vi "Get SMO HELP.vi"(8 "error in (no error)":errorcluster, 10 "Command":string, 11 "Instrument in":refnum<class "Instrument.lvclass">) -> (0 "error out":errorcluster, 2 "output cluster":T1, 3 "Instrument out":refnum<class "Instrument.lvclass">)   [LabVIEW 2019, in "Instrument.lvclass"]
uses:
  Instrument.lvclass
  Help/typedefs/Help--cluster.ctl
  Typedefs/Instrument.Commands--Enum.ctl
  Typedefs/Instrument.IDN--cluster.ctl
  Help/Help.lvclass
  <vilib>/JKI/JKI SMO/SMO/SMO.lvclass
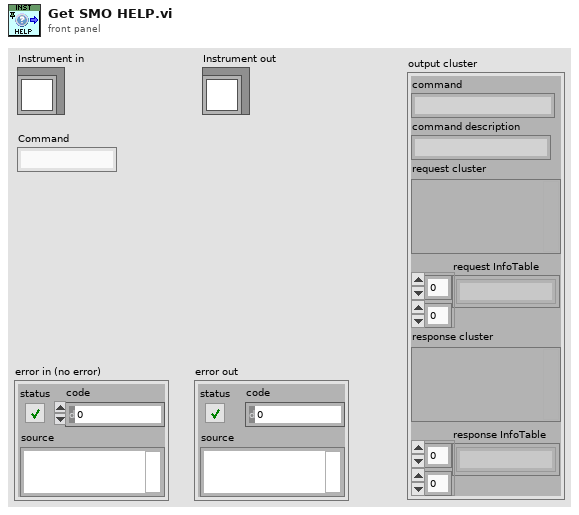
[diagram p1: front panel]
types:
  T1 = typedef "Help.lvclass/Help--cluster.ctl" = cluster{"command":string, "command description":string, "request cluster":variant, "request InfoTable":string[][], "response cluster":variant, "response InfoTable":string[][]}
  T2 = typedef "Instrument.lvclass/Instrument.Commands--Enum.ctl" = enum16{"ACK", "HELP", "IDN", "getAll", "getAllData"}
  T3 = typedef "Instrument.lvclass/Instrument.IDN--cluster.ctl" = cluster{"vendor":string, "model":string, "serial":string, "firmware":string}
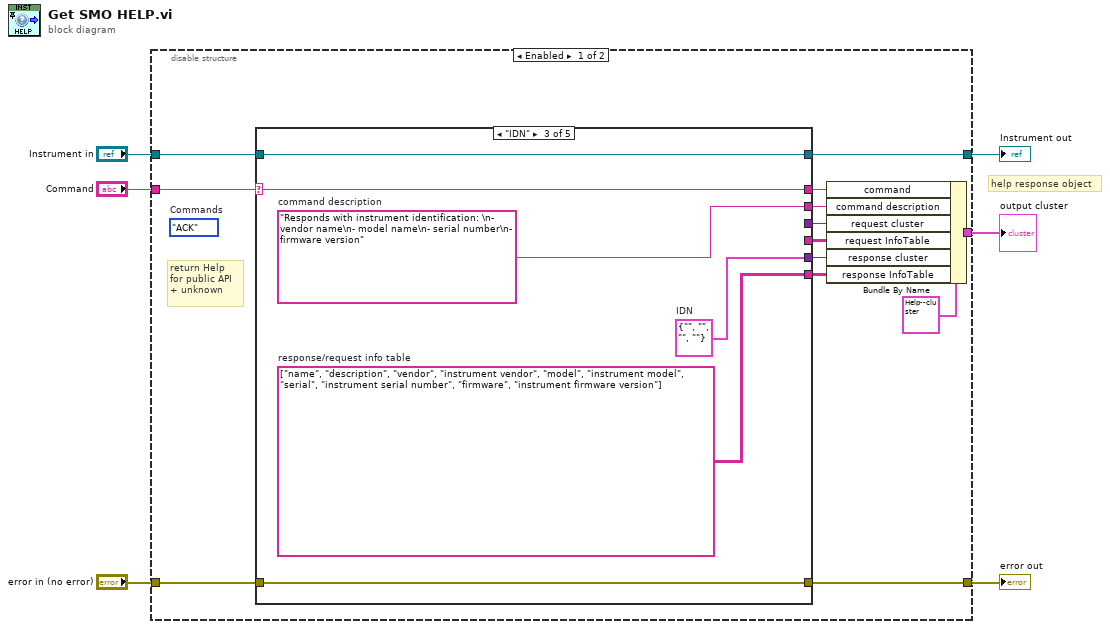
[diagram p0: block diagram]
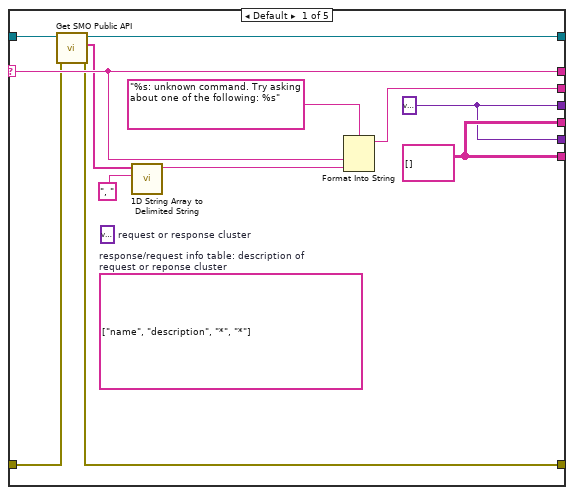
[diagram p2: hidden frame]
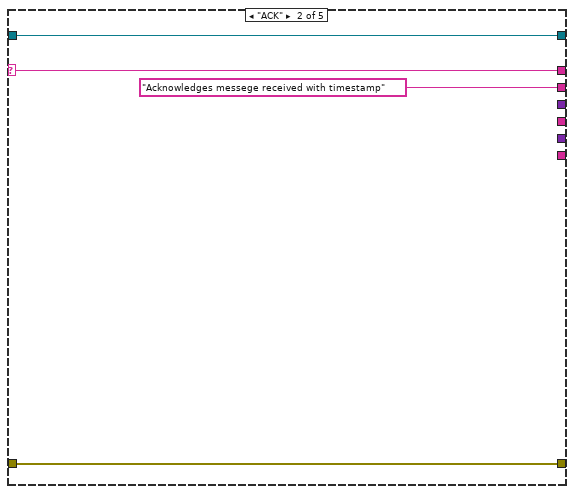
[diagram p3: hidden frame]
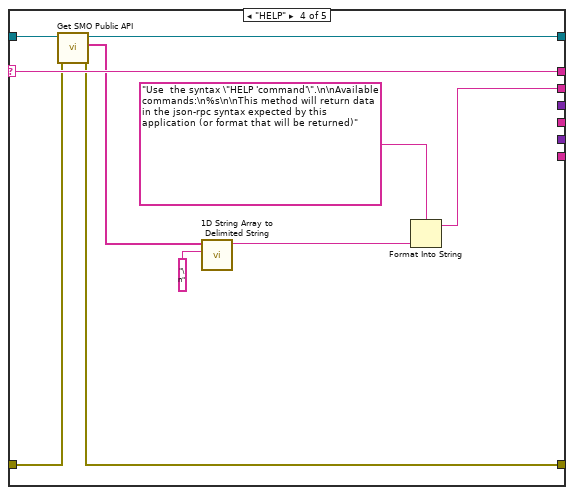
[diagram p4: hidden frame]
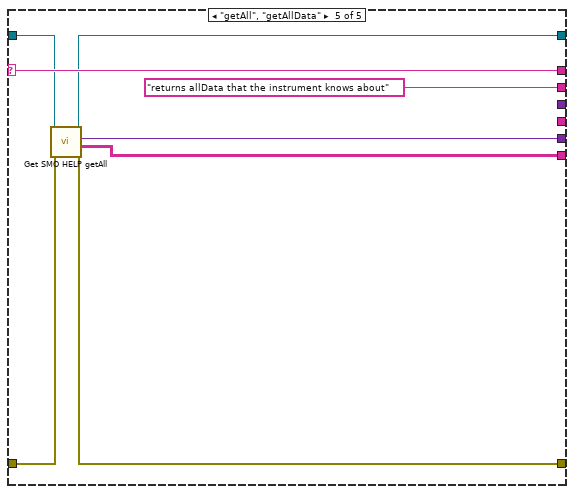
[diagram p5: hidden frame]
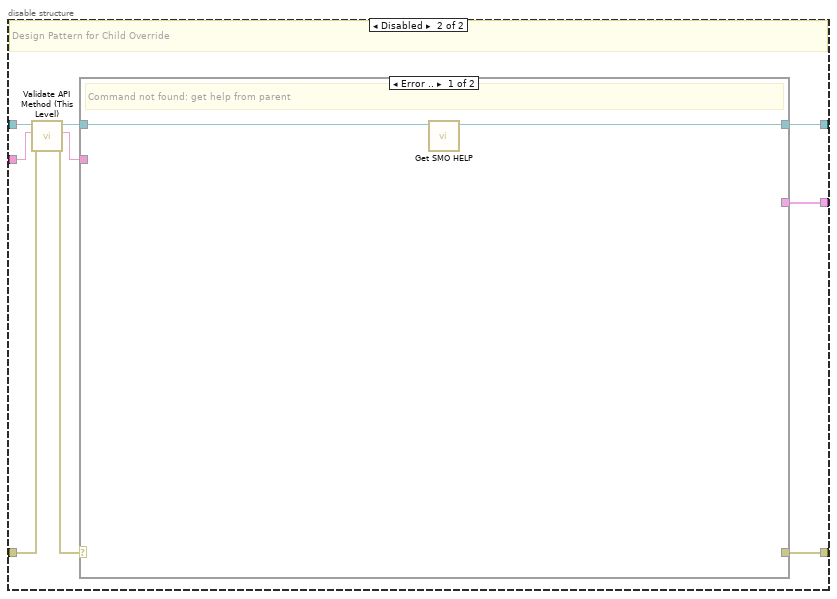
[diagram p6: hidden frame]
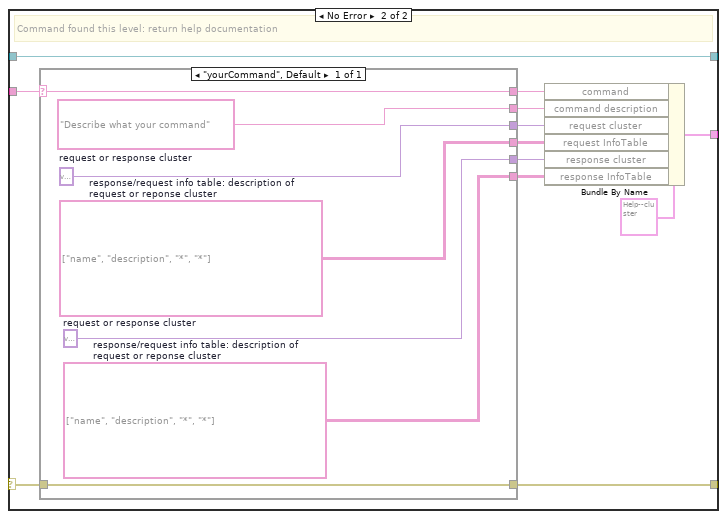
[diagram p7: hidden frame]
diagram:
  # "help response object"
  n1 = disable-structure shown="Enabled" {
    disable-tunnel: [w19 w68] -> w6
    disable-tunnel: "Instrument in" -> [w18 w65]
    disable-tunnel: "error in (no error)" -> [w17 w63]
    disable-tunnel: [w13 w67] -> w3
    disable-tunnel: [w8 w66] -> w2
    disable-tunnel: "Command" -> [w7 w64]
    frame Enabled {
      (unwired) Instrument.Commands--Enum."ACK"  # Commands
      # "return Help\nfor public API\n+ unknown"
      n2 = case shown="\"IDN\"" w7 {
        selector: w7 -> [w27 w33 w40 w48 w58]
        tunnel: w17 -> [w23 w35 w36 w43 w57]
        tunnel: [w24 w35 w36 w44 w56] -> w13
        tunnel: [w29 "Acknowledges messege received with timestamp" w41 w47 "returns allData that the instrument knows about"] -> w15
        tunnel: [w20 _ _ _ _] -> w14
        tunnel: [w21 _ _ _ _] -> w10
        tunnel: [w21 _ w37 _ w52] -> w12
        tunnel: [w20 _ w38 _ w55] -> w11
        tunnel: [w27 w33 w40 w48 w58] -> w16
        tunnel: w18 -> [w26 w32 w39 w46 w53]
        tunnel: [w22 w32 w39 w42 w54] -> w19
        frame Default {
          (unwired) variant  # request or response cluster
          (unwired) string[][] [["name", "description"], ["*", "*"]]  # response/request info table: description of request or reponse cluster
          w20 = variant ("response cluster")
          w21 = string[][] [] ("response/request info table")
          n3 = call-dynamic "Get SMO Public API.vi"("error in (no error)"=w23, "Instrument in"=w26) -> ("error out"=w24:errorcluster, "commands"=w25:string[], "Instrument out"=w22:refnum<class "Instrument.lvclass">)  [unwired: 7 in]
          n4 = call <vilib>:"1D String Array to Delimited String.vi"("delimiter"=", ", "string array"=w25) -> ("delimited string"=w30:string)  [unwired: 9 in]
          n5 = Format Into String(format string="%s: unknown command. Try asking about one of the following: %s", w27, w30) -> (resulting string=w29:string)  [unwired: 2 in, 1 out]
        }
        frame "ACK" {
        }
        frame "IDN" {
          w37 = string[][] [["name", "description"], ["vendor", "instrument vendor"], ["model", "instrument model"], ["serial", "instrument serial number"], ["firmware", "instrument firmware version"]]  # response/request info table
          w38 = T3 {"vendor"="", "model"="", "serial"="", "firmware"=""}  # IDN
          w41 = "Responds with instrument identification: \n- vendor name\n- model name\n- serial number\n- firmware version"  # command description
        }
        frame "HELP" {
          n6 = call-dynamic "Get SMO Public API.vi"("error in (no error)"=w43, "Instrument in"=w46) -> ("error out"=w44:errorcluster, "commands"=w45:string[], "Instrument out"=w42:refnum<class "Instrument.lvclass">)  [unwired: 7 in]
          n7 = call <vilib>:"1D String Array to Delimited String.vi"("delimiter"="\n", "string array"=w45) -> ("delimited string"=w51:string)  [unwired: 9 in]
          n8 = Format Into String(format string="Use  the syntax \"HELP 'command'\".\n\nAvailable commands:\n%s\n\nThis method will return data in the json-rpc syntax expected by this application (or format that will be returned)", w51) -> (resulting string=w47:string)  [unwired: 2 in, 1 out]
        }
        frame "getAll", "getAllData" {
          n9 = call-dynamic "Get SMO HELP getAll.vi"("error in (no error)"=w57, "Instrument in"=w53) -> ("error out"=w56:errorcluster, "response info table"=w52:string[][], "response cluster"=w55:variant, "Instrument out"=w54:refnum<class "Instrument.lvclass">)  [unwired: 6 in]
        }
      }
      n10 = Bundle By Name(cluster=T1 {"command"="", "command description"="", "request cluster"=variant, "request InfoTable"=[], "response cluster"=variant, "response InfoTable"=[]} ("Help"), "command"=w16, "command description"=w15, "request cluster"=w14, "request InfoTable"=w10, "response cluster"=w11, "response InfoTable"=w12) -> (w8:T1)
    }
    frame Disabled {
      # "Design Pattern for Child Override"
      n11 = call "Validate API Method (This Level).vi"("error in (no error)"=w63, "Command in"=w64, "Instrument in"=w65) -> ("error out"=w62:errorcluster, "command out"=w60:string, "Instrument out"=w61:refnum<class "Instrument.lvclass">)  [unwired: 6 in]
      n12 = case shown="Error .." w62 {
        selector: w62 -> [_ w77]
        tunnel: w61 -> [w69 w82]
        tunnel: [w69 w82] -> w68
        tunnel: [_ w76] -> w67
        tunnel: [w70 w81] -> w66
        tunnel: w60 -> [_ w79]
        frame Error {
          # "Command not found: get help from parent"
          n13 = call-parent "Get SMO HELP.vi"() -> ()  [unwired: 1 in]
        }
        frame No Error {
          # "Command found this level: return help documentation"
          n14 = case shown="\"yourCommand\", Default" w79 {
            selector: w79 -> [w89]
            tunnel: [w89] -> w78
            tunnel: w77 -> [w88]
            tunnel: [w88] -> w76
            tunnel: ["Describe what your command"] -> w75
            tunnel: [w86] -> w74
            tunnel: [w85] -> w73
            tunnel: [w84] -> w72
            tunnel: [w83] -> w71
            frame "yourCommand", Default {
              w86 = variant  # request or response cluster
              w85 = string[][] [["name", "description"], ["*", "*"]]  # response/request info table: description of request or reponse cluster
              w84 = variant  # request or response cluster
              w83 = string[][] [["name", "description"], ["*", "*"]]  # response/request info table: description of request or reponse cluster
            }
          }
          n15 = Bundle By Name(cluster=T1 {"command"="", "command description"="", "request cluster"=variant, "request InfoTable"=[], "response cluster"=variant, "response InfoTable"=[]} ("Help"), "command"=w78, "command description"=w75, "request cluster"=w74, "request InfoTable"=w73, "response cluster"=w72, "response InfoTable"=w71) -> (w81:T1)
        }
      }
    }
  }
  "Instrument out" <- w6
  "output cluster" <- w2
  "error out" <- w3
